vi "getBentStyle.vi"(0 "reference":refnum<class "BentStyle.lvclass">, 5 "error in (no error)":errorcluster) -> (14 "reference out":refnum<class "BentStyle.lvclass">, 15 "bentStyle":T1, 19 "error out":errorcluster)   [LabVIEW 2020, in "BentStyle.lvclass"]
doc: "Get Bent style"
uses:
  <resource>/Framework/Providers/Open_GDS/UML/BentStyle_class/BentStyle.lvclass
  <resource>/Framework/Providers/Open_GDS/UML/BentStyle_class/BentStyleType.ctl
  <resource>/Framework/Providers/Open_GDS/UML/BentStyle_class/BentStyle.lvclass/BentStyle.ctl
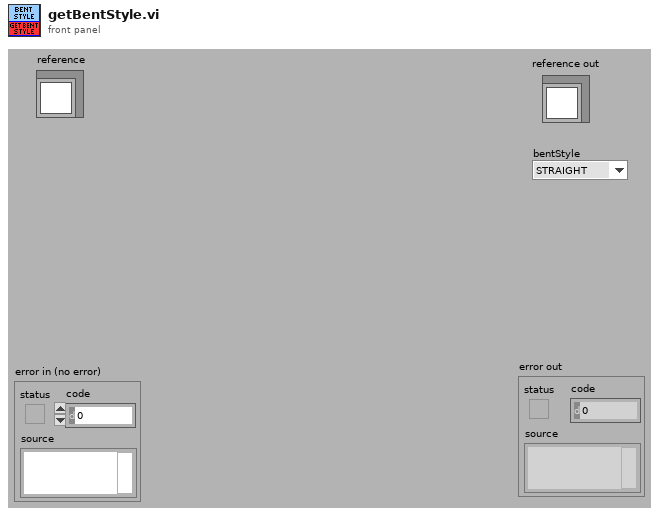
[diagram p1: front panel]
types:
  T1 = typedef "BentStyle.lvclass/BentStyleType.ctl" = enum16{"STRAIGHT", "HV", "VH", "HVH", "VHV", "ARC"}
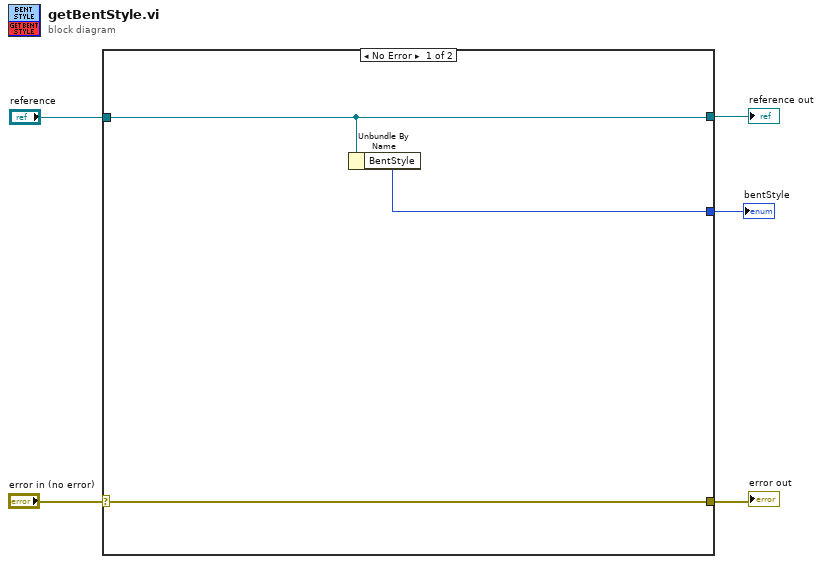
[diagram p0: block diagram]
diagram:
  n1 = case shown="No Error" "error in (no error)" {
    selector: "error in (no error)" -> [w6 w9]
    tunnel: "reference" -> [w8 w10]
    tunnel: [w6 w9] -> w3
    tunnel: [w8 w10] -> w2
    tunnel: [w7 _] -> w1
    frame No Error {
      n2 = Unbundle By Name(w8) -> ("BentStyle"=w7:T1)
    }
    frame Error {
    }
  }
  "reference out" <- w2
  "error out" <- w3
  "bentStyle" <- w1
